vi "Open Dialog VI.vi"(8 "error in":errorcluster, 9 "Windows title":string, 10 "ref for signalling":refnum<vi>, 11 "vi path":path=path "Display Settings.vi") -> (0 "error out":errorcluster)   [LabVIEW 2020, in "POLARIS IMAQ Display.xctl"]
uses:
  POLARIS IMAQ Display.xctl
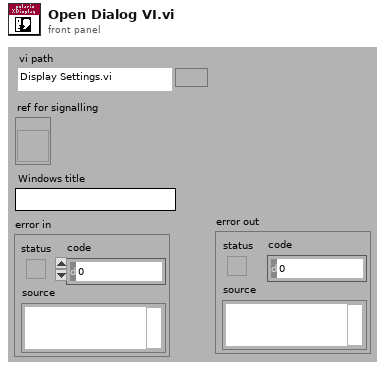
[diagram p1: front panel]
types:
  T1 = enum32{"Invalid", "Standard", "Closed", "Hidden", "Minimized", "Maximized"}
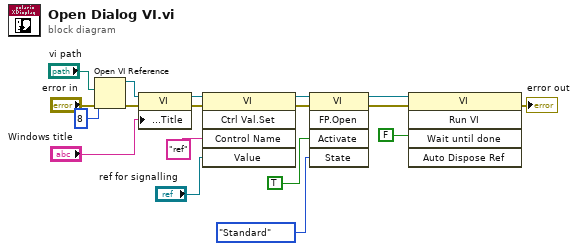
[diagram p0: block diagram]
diagram:
  n1 = Open VI Reference(vi path="vi path", options=8, error in (no error)="error in") -> (vi reference=w13:refnum<vi>, error out=w14:errorcluster)  [unwired: 3 in]
  n2 = property class="VI"(reference=w13, error in=w14, "Front Panel.Title"="Windows title") -> (reference out=w4:refnum<vi>, error out=w16:errorcluster)
  n3 = invoke class="VI" method="Ctrl Val.Set"(reference=w4, error in=w16, "Control Name"="ref", "Value"="ref for signalling") -> (reference out=w17:refnum<vi>, error out=w18:errorcluster)  [unwired: 1 in, 3 out]
  n4 = invoke class="VI" method="FP.Open"(reference=w17, error in=w18, "Activate"=TRUE ("Activate?"), "State"=T1."Standard") -> (reference out=w9:refnum<vi>, error out=w10:errorcluster)  [unwired: 1 in, 3 out]
  n5 = invoke class="VI" method="Run VI"(reference=w9, error in=w10, "Wait until done"=FALSE ("Wait Until Done")) -> (error out=→"error out":errorcluster)  [unwired: 2 in, 4 out]
